vi "Register Modules in UI Manager--helper.vi"(7 "Application in":refnum<vi>, 8 "error in (no error)":errorcluster, 10 "New Modules":path[](array[path]), 11 "Modules IN":path[](array[path])) -> (0 "error out":errorcluster, 3 "Modules OUT":path[](array[path]))   [LabVIEW 2022 SP3, in "UI Manager.lvlib"]
doc: "____\nHAMPEL SOFTWARE ENGINEERING v2.6.0 (2023-12-19 10:54)"
uses:
  UI Manager.lvlib
  Libraries/hse-libraries/Source/hse-application/hse-application.lvclass/hse-application.ctl
  Libraries/hse-libraries/Source/hse-application/HSE Application not initialized--error.vi
  <vilib>/Utility/error.llb/Clear Errors.vi
  Libraries/hse-libraries/Source/hse-application/hse-application__GetSingleton.vi
  <vilib>/Utility/sysdir.llb/Get System Directory.vi
  <vilib>/Utility/error.llb/Error Cluster From Error Code.vi
  Libraries/hse-libraries/Source/hse-dqmh/hse-dqmh-dynamicrequesters.lvlib
  Libraries/hse-libraries/Source/hse-application/hse-application.lvclass
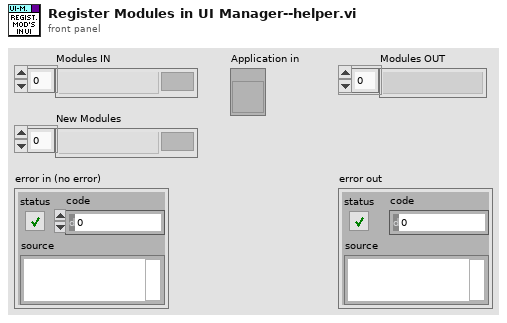
[diagram p1: front panel]
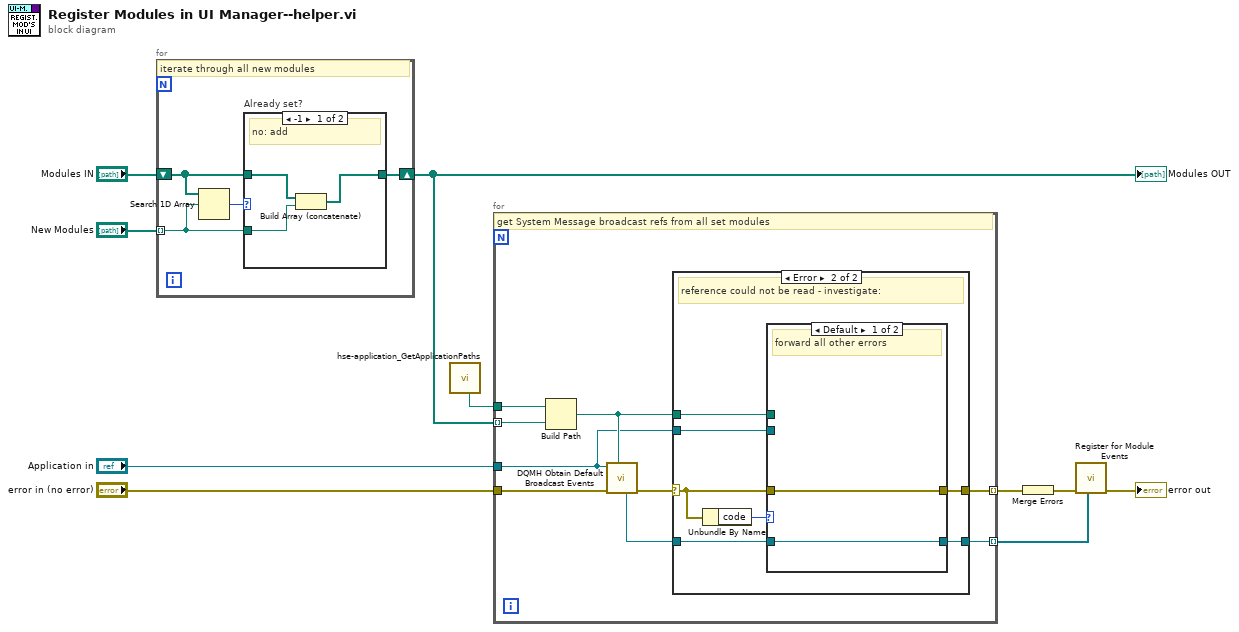
[diagram p0: block diagram]
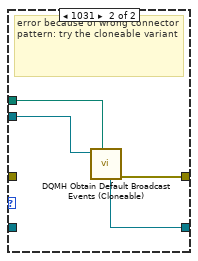
[diagram p4: hidden frame]
diagram:
  n1 = for {
    tunnel: "New Modules" -> [w11] mode=indexing
    shift-right: [w13] -> w2
    shift-left: "Modules IN" -> [w12]
    # "iterate through all new modules"
    n2 = Search 1D Array(1D array=w12, element=w11) -> (index of element=w14:i32)  [unwired: 1 in]
    n3 = case "Already set?" shown="-1" w14 {
      tunnel: [w15 w18] -> w13
      tunnel: w12 -> [w16 w18]
      tunnel: w11 -> [w17 _]
      frame -1 {
        # "no: add"
        n4 = Build Array (concatenate)(w16, w17) -> (w15:path[])
      }
      frame Default {
        # "yes: do nothing"
      }
    }
  }
  "Modules OUT" <- w2
  n5 = call "hse-application_GetApplicationPaths.vi"() -> ("Application Base Path"=w1:path)  [unwired: 5 in, 6 out]
  n6 = for {
    tunnel: w2 -> [w27] mode=indexing
    tunnel: w1 -> [w26]
    tunnel: "error in (no error)" -> [w25]
    tunnel: [w22] -> w4 mode=indexing
    tunnel: "Application in" -> [w19]
    tunnel: [w21] -> w7 mode=indexing
    # "get System Message broadcast refs from all set modules"
    n7 = Build Path(base path=w26, name or relative path=w27) -> (appended path=w20:path)
    n8 = call "DQMH Obtain Default Broadcast Events.vi"("Module Disk Path"=w20, "error in (no error)"=w25, "Application reference"=w19) -> ("error out"=w24:errorcluster, "System Message"=w23:refnum<user-event>)  [unwired: 3 in, 4 out]
    n9 = case shown="Error" w24 {
      selector: w24 -> [w29 w31]
      tunnel: w23 -> [w28 w30]
      tunnel: [w29 w36] -> w22
      tunnel: [w28 w33] -> w21
      tunnel: w20 -> [_ w35]
      tunnel: w19 -> [_ w34]
      frame No Error {
        # "broadcast reference read successfully"
      }
      frame Error {
        # "reference could not be read - investigate:"
        n10 = Unbundle By Name(w31) -> ("code"=w32:i32)
        n11 = case shown="Default" w32 {
          tunnel: [w37 w42] -> w36
          tunnel: w35 -> [_ w41]
          tunnel: w34 -> [_ w40]
          tunnel: [w38 w39] -> w33
          tunnel: w31 -> [w37 _]
          tunnel: w30 -> [w38 _]
          frame Default {
            # "forward all other errors"
          }
          frame 1031 {
            # "error because of wrong connector pattern: try the cloneable variant"
            n12 = call "DQMH Obtain Default Broadcast Events (Cloneable).vi"("Module Disk Path"=w41, "Application reference"=w40) -> ("error out"=w42:errorcluster, "System Message"=w39:refnum<user-event>)  [unwired: 4 in, 4 out]
          }
        }
      }
    }
  }
  n13 = Merge Errors(w4) -> (w6:errorcluster)
  n14 = call "Register for Module Events.vi"("System Messages"=w7, "error in (no error)"=w6) -> ("error out"=→"error out":errorcluster)  [unwired: 9 in]
